vi "MT Generate Bits (User Defined).vi"(0 "total bits (128)":i32=128, 2 "user base bit pattern":i8[](array[numeric]), 11 "error in (no error)":errorcluster, 13 "reset? (T)":bool=TRUE) -> (4 "output bit stream":i8[](array[numeric]), 15 "error out":errorcluster)   [LabVIEW 2020, in "niDMT.lvlib"]
doc: "This polymorphic instance generates bit sequences based on a pattern that you specify. The toolkit repeats the selected pattern until it generates the number of bits that you specify."
uses:
  <vilib>/addons/Modulation/niDMT.lvlib
  <vilib>/addons/Modulation/niAMT.lvlib
panel:
  # "User mode"
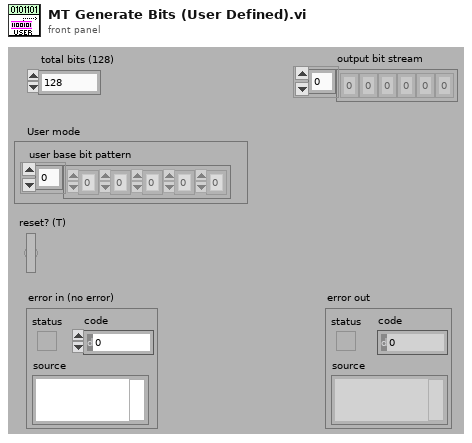
[diagram p1: front panel]
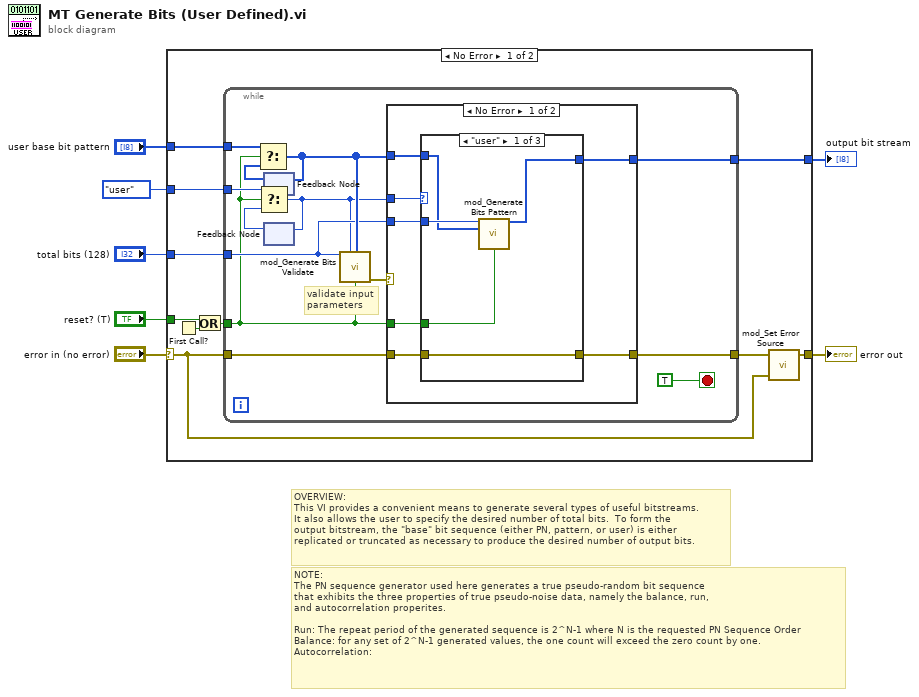
[diagram p0: block diagram]
diagram:
  # "OVERVIEW:\nThis VI provides a convenient means to generate several types of useful bitstreams.\nIt also allows the user to specify the desired number of total bits.  To form the\noutput bitstream, the \"base\" bit sequence (either PN, pattern, or user) is either\nreplicated or truncated as necessary to produce the desired number of output bits."
  # "NOTE:\nThe PN sequence generator used here generates a true pseudo-random bit sequence\nthat exhibits the three properties of true pseudo-noise data, namely the balance, run,\nand autocorrelation properites.\n\nRun: The repeat period of the generated sequence is 2^N-1 where N is the requested PN Sequence Order\nBalance: for any set of 2^N-1 generated values, the one count will exceed the zero count by one.\nAutocorrelation:"
  n1 = case shown="No Error" "error in (no error)" {
    selector: "error in (no error)" -> [w8 w46]
    tunnel: [w12 w46] -> w6
    tunnel: "total bits (128)" -> [w16 _]
    tunnel: enum16{"PN", "pattern", "user"}."user" ("mode (PN)") -> [w15 _]
    tunnel: "reset? (T)" -> [w10 _]
    tunnel: [w17 i8[] []] -> w1
    tunnel: "user base bit pattern" -> [w14 _]
    frame No Error {
      n2 = First Call?() -> (First Call?: T/F=w11:bool)
      n3 = Or(x=w10, y=w11) -> (x .or. y?=w9:bool)
      n4 = while {
        tunnel: [w30] -> w17
        tunnel: w16 -> [w22]
        tunnel: w15 -> [w21]
        tunnel: w14 -> [w25]
        tunnel: [w28] -> w13
        tunnel: w8 -> [w27]
        tunnel: w9 -> [w20]
        stop <- TRUE stop-if-true
        # "validate input parameters"
        n5 = feedback #1() -> (w26:i8[])  [unwired: 1 out]
        n6 = Select(t=w25, s=w20, f=w26) -> (s? t:f=w23:i8[])
        n7 = feedback-in #1(w23) -> ()
        n8 = feedback #2() -> (w19:enum16{"PN", "pattern", "user"})  [unwired: 1 out]
        n9 = Select(t=w21, s=w20, f=w19) -> (s? t:f=w18:enum16{"PN", "pattern", "user"})
        n10 = feedback-in #2(w18) -> ()
        n11 = call <vilib>:"mod_Generate Bits Validate.vi"("Total Bits"=w22, "Mode (PN)"=w18, "User Base Bit Pattern"=w23, "reset?"=w20) -> ("error out"=w29:errorcluster)  [unwired: 2 in, 9 out]
        n12 = case shown="No Error" w29 {
          selector: w29 -> [_ w44]
          tunnel: w27 -> [w37 _]
          tunnel: [w36 w44] -> w28
          tunnel: w18 -> [w35 _]
          tunnel: [w34 i8[] [] ("Output Data Bit Sequence")] -> w30
          tunnel: w22 -> [w33 _]
          tunnel: w20 -> [w32 _]
          tunnel: w23 -> [w31 _]
          frame No Error {
            n13 = case shown="\"user\"" w35 {
              tunnel: w37 -> [w42 _ _]
              tunnel: [w42 _ _] -> w36
              tunnel: w31 -> [w39 _ _]
              tunnel: [w38 _ _] -> w34
              tunnel: w33 -> [w41 _ _]
              tunnel: w32 -> [w40 _ _]
              frame "user" {
                n14 = call <vilib>:"mod_Generate Bits Pattern.vi"("Total Bits"=w41, "Reset? (T)"=w40, "User Base Bit Pattern"=w39) -> ("Output Bit Stream"=w38:i8[])  [unwired: 12 out]
              }
              frame "pattern" {
              }
              frame "PN" {
              }
            }
          }
          frame Error {
            # "Invalid inputs - generate error"
          }
        }
      }
      n15 = call <vilib>:"mod_Set Error Source.vi"("initial error in (no error)"=w8, "final error in (no error)"=w13) -> ("error out"=w12:errorcluster)  [unwired: 3 out]
    }
    frame Error {
    }
  }
  "error out" <- w6
  "output bit stream" <- w1
